vi "Write Tracer-V Queue.vi"(8 "error in (no error)":errorcluster, 10 "TraceMessage Queue":refnum<queue>, 11 "Tracer-V in":refnum<class "Tracer-V.lvclass">) -> (0 "error out":errorcluster, 3 "Tracer-V out":refnum<class "Tracer-V.lvclass">)   [LabVIEW 2013, in "Tracer-V.lvclass"]
uses:
  Tracer-V.lvclass
  Logical Systems/TraceMessage/Trace.lvclass
  Tracer-V.lvclass/Tracer-V.ctl
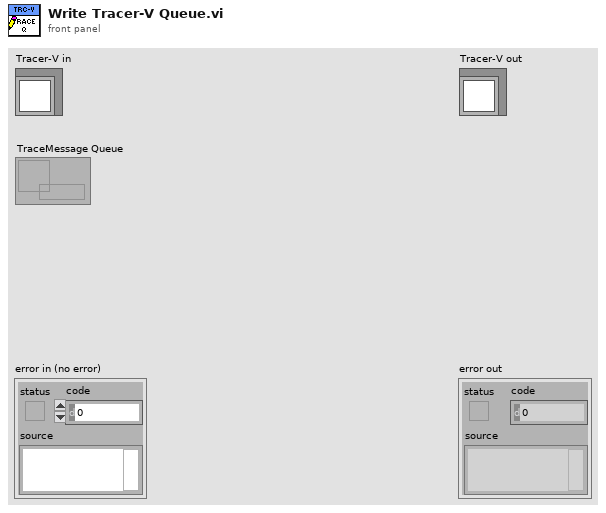
[diagram p1: front panel]
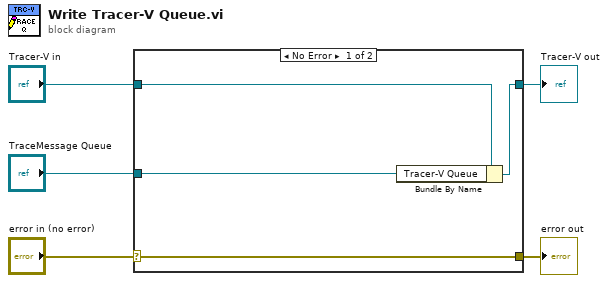
[diagram p0: block diagram]
diagram:
  n1 = case shown="No Error" "error in (no error)" {
    selector: "error in (no error)" -> [w9 w10]
    tunnel: [w9 w10] -> w4
    tunnel: [w7 w11] -> w2
    tunnel: "Tracer-V in" -> [w8 w11]
    tunnel: "TraceMessage Queue" -> [w6 _]
    frame No Error {
      n2 = Bundle By Name(cluster=w8, "Tracer-V Queue"=w6) -> (w7:refnum<class "Tracer-V.lvclass">)
    }
    frame Error {
    }
  }
  "error out" <- w4
  "Tracer-V out" <- w2
